vi "Forward Generic Broadcasts to Network.vi"(8 "error in (no error)":errorcluster, 9 "Network Broadcast Params":T2, 10 "Generic Broadcast Events":T1, 11 "Module ID":i32=-1) -> (0 "error out":errorcluster)   [LabVIEW 2020, in "GenNet-Server.lvlib"]
doc: "Enables forwarding of the callers <b>Generic Broadcast Events</b> to the network via UDP as set in the <b>Network Broadcast Params</b>.\n____\nHAMPEL SOFTWARE ENGINEERING v3.8.0 (2023-12-18 14:41)"
uses:
  GenNet-Server.lvlib
  UDP Broadcasting/Network Broadcast Params.ctl
  UDP Broadcasting/Generic Broadcasts.ctl
  hse-dqmh/Dynamic Requesters/Singleton/Status Updated Argument--cluster.ctl
  hse-dqmh/Dynamic Requesters/Singleton/Error Reported Argument--cluster.ctl
  hse-dqmh/Dynamic Requesters/Singleton/Get Module Execution Status Argument--cluster.ctl
  hse-dqmh/Dynamic Requesters/Singleton/Stop Argument--cluster.ctl
  hse-dqmh/Controls/System Message Argument--cluster.ctl
  hse-dqmh/Controls/System Message Source.ctl
  Forward Generic Broadcasts to Network Argument--cluster.ctl
  hse-gennet.lvlib
  hse-dqmh/hse-dqmh.lvlib
  hse-dqmh/hse-dqmh-dynamicrequesters.lvlib
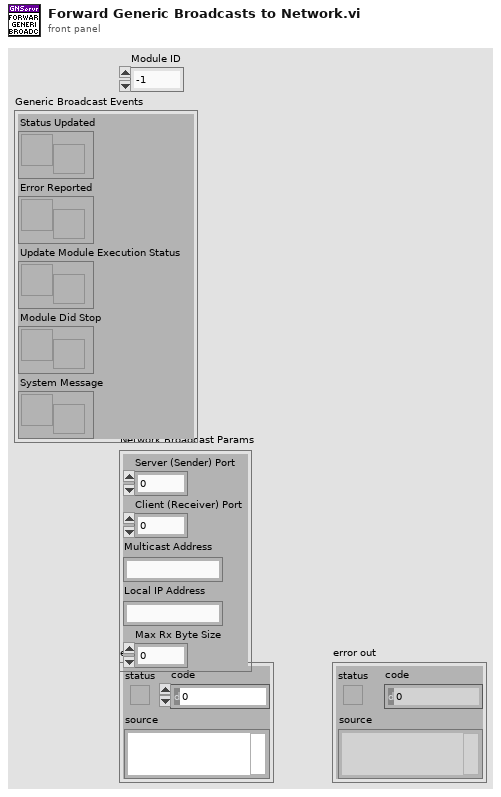
[diagram p1: front panel]
types:
  T1 = typedef "hse-gennet.lvlib/Generic Broadcasts.ctl" = cluster{"Status Updated":refnum<user-event>, "Error Reported":refnum<user-event>, "Update Module Execution Status":refnum<user-event>, "Module Did Stop":refnum<user-event>, "System Message":refnum<user-event>}
  T2 = typedef "hse-gennet.lvlib/Network Broadcast Params.ctl" = cluster{"Server (Sender) Port":u16, "Client (Receiver) Port":u16, "Multicast Address":string, "Local IP Address":string, "Max Rx Byte Size":i32}
  T3 = typedef "GenNet-Server.lvlib/Forward Generic Broadcasts to Network Argument--cluster.ctl" = cluster{"Module ID":i32, "Generic Broadcast Events":T1, "Network Broadcast Params":T2}
  T4 = typedef "GenNet-Server.lvlib/Request Events--cluster.ctl" = cluster{"Stop Module":refnum<user-event>, "Show Panel":refnum<user-event>, "Hide Panel":refnum<user-event>, "Show Diagram":refnum<user-event>, "Get Module Execution Status":refnum<user-event>, "Forward Generic Broadcasts to Network":refnum<user-event>}
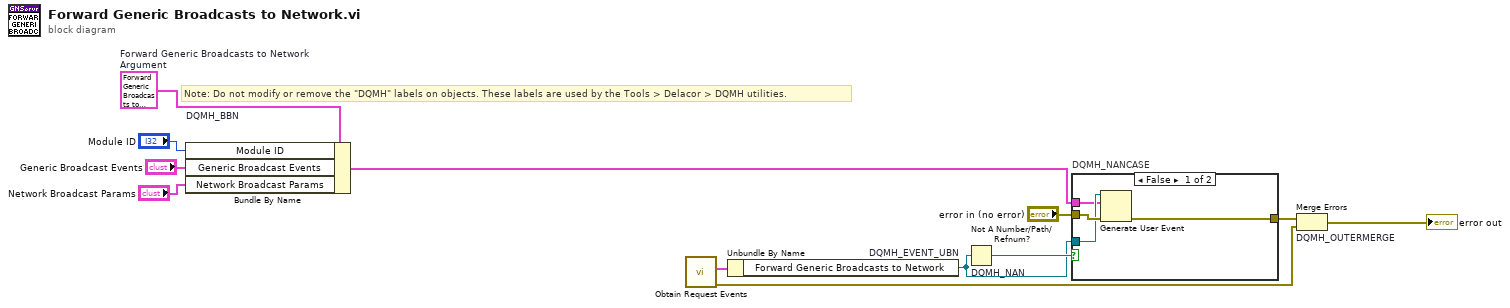
[diagram p0: block diagram]
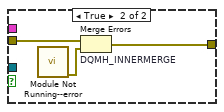
[diagram p2: hidden frame]
diagram:
  w2 = T3 {"Module ID"=-1, "Generic Broadcast Events"={"Status Updated"=refnum, "Error Reported"=refnum, "Update Module Execution Status"=refnum, "Module Did Stop"=refnum, "System Message"=refnum}, "Network Broadcast Params"={"Server (Sender) Port"=0, "Client (Receiver) Port"=0, "Multicast Address"="", "Local IP Address"="", "Max Rx Byte Size"=0}}  # Forward Generic Broadcasts to Network Argument
  # "Note: Do not modify or remove the \"DQMH\" labels on objects. These labels are used by the Tools > Delacor > DQMH utilities."
  n1 = Bundle By Name "DQMH_BBN"(cluster=w2, "Module ID"="Module ID", "Generic Broadcast Events"="Generic Broadcast Events", "Network Broadcast Params"="Network Broadcast Params") -> (w10:T3)
  n2 = call "Obtain Request Events.vi"() -> ("error out"=w4:errorcluster, "GenNet-Server Request Events"=w3:T4)  [unwired: 10 in]
  n3 = Unbundle By Name "DQMH_EVENT_UBN"(w3) -> ("Forward Generic Broadcasts to Network"=w8:refnum<user-event>)
  n4 = Not A Number/Path/Refnum? "DQMH_NAN"(number/path/refnum=w8) -> (NaN/Path/Refnum?=w9:bool)
  n5 = case "DQMH_NANCASE" shown="False" w9 {
    tunnel: "error in (no error)" -> [w16 w19]
    tunnel: [w15 w18] -> w7
    tunnel: w8 -> [w14 _]
    tunnel: w10 -> [w13 _]
    frame False {
      n6 = Generate User Event(user event=w14, event data cluster=w13, error in=w16) -> (error out=w15:errorcluster)  [unwired: 1 in, 1 out]
    }
    frame True {
      n7 = call "Module Not Running--error.vi"() -> ("error out"=w17:errorcluster)  [unwired: 11 in]
      n8 = Merge Errors "DQMH_INNERMERGE"(w19, w17) -> (w18:errorcluster)
    }
  }
  n9 = Merge Errors "DQMH_OUTERMERGE"(w7, w4) -> (→"error out":errorcluster)
